vi "hash action stack.vi"(6 "init size":i32=50, 7 "stack action":T2, 8 "hash action list":T1[](array[typedef]), 9 "hash action":T1, 11 "command stack":T1[](array[typedef])) -> (1 "cursor window action out":T1, 2 "stack is empty ?":bool, 3 "command stack out":T1[](array[typedef]))   [LabVIEW 2017]
uses:
  stack action -- control.ctl
  hash action control.ctl
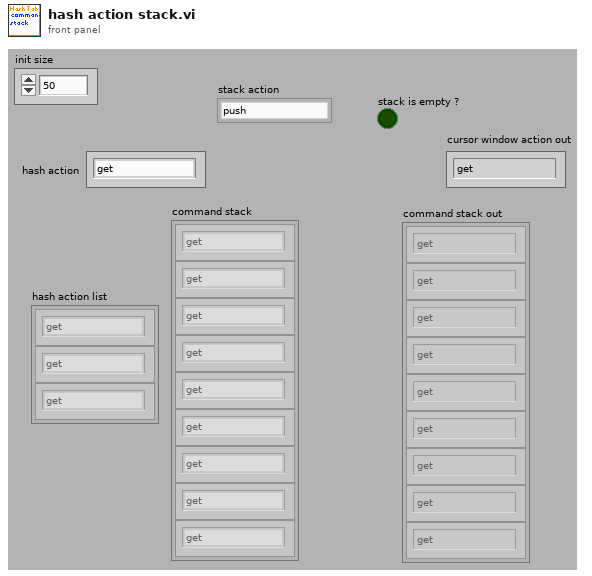
[diagram p1: front panel]
types:
  T1 = typedef "hash action control.ctl" = enum16{"get", "new", "--void", "delete", "delete all", "set", "--delete if exists", "--create if not there", "list keys", "index forw", "index back", "check", "index set", "find key"}
  T2 = typedef "stack action -- control.ctl" = enum16{"push", "pop", "check", "init"}
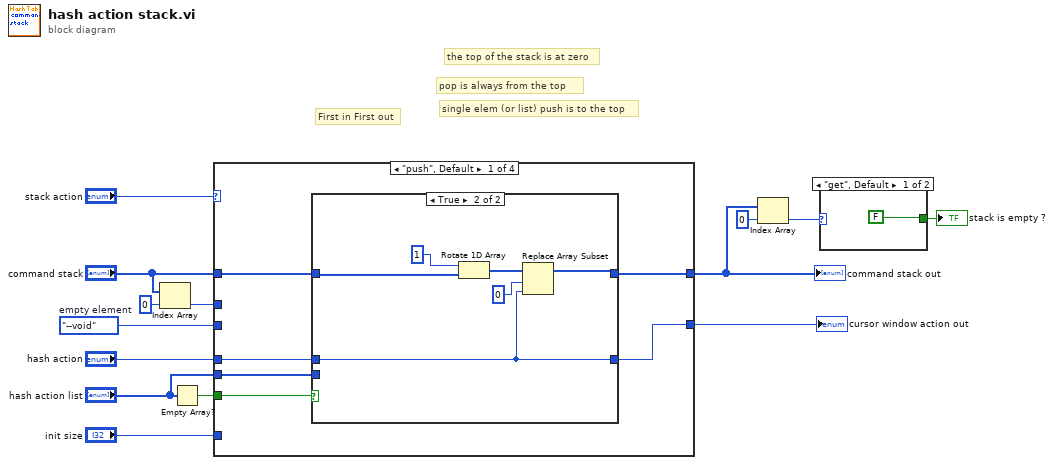
[diagram p0: block diagram]
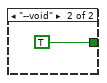
[diagram p2: hidden frame]
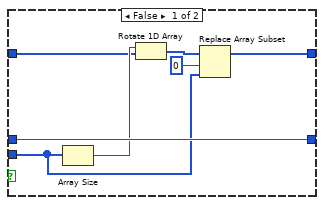
[diagram p3: hidden frame]
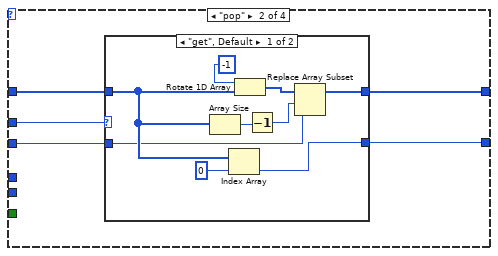
[diagram p4: hidden frame]
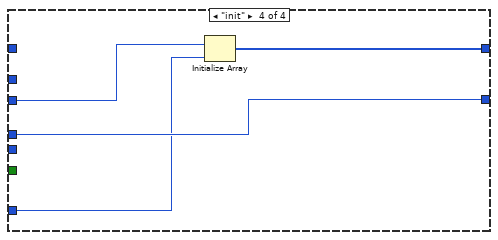
[diagram p7: hidden frame]
diagram:
  w2 = hash_action_control."--void"  # empty element
  # "single elem (or list) push is to the top"
  # "pop is always from the top"
  # "First in First out"
  # "the top of the stack is at zero"
  n1 = Index Array(array="command stack", index=0) -> (element=w6:T1)
  n2 = Empty Array?(array="hash action list") -> (empty?=w11:bool)
  n3 = case shown="\"push\", Default" "stack action" {
    tunnel: w6 -> [_ w38 _ _]
    tunnel: [w17 w37 w51 w55] -> w12
    tunnel: "hash action" -> [w20 _ w51 w55]
    tunnel: w11 -> [w19 _ _ _]
    tunnel: "hash action list" -> [w18 _ _ _]
    tunnel: "command stack" -> [w16 w36 w50 _]
    tunnel: [w15 w35 w50 w52] -> w4
    tunnel: w2 -> [_ w34 _ w54]
    tunnel: "init size" -> [_ _ _ w53]
    frame "push", Default {
      n4 = case shown="True" w19 {
        tunnel: w20 -> [w27 w31]
        tunnel: w18 -> [w21 _]
        tunnel: [w27 w31] -> w17
        tunnel: w16 -> [w23 w29]
        tunnel: [w22 w28] -> w15
        frame False {
          n5 = Array Size(array=w21) -> (size(s)=w26:i32)
          n6 = Rotate 1D Array(1:w23, 2:w26) -> (0:w25:T1[])
          n7 = Replace Array Subset(array=w25, new element=w21, index=0) -> (w22:T1[])
        }
        frame True {
          n8 = Rotate 1D Array(1:w29, 2:1) -> (0:w33:T1[])
          n9 = Replace Array Subset(array=w33, new element=w31, index=0) -> (w28:T1[])
        }
      }
    }
    frame "pop" {
      n10 = case shown="\"get\", Default" w38 {
        tunnel: [w45 w48] -> w37
        tunnel: w36 -> [w44 w49]
        tunnel: [w42 w49] -> w35
        tunnel: w34 -> [w39 w48]
        frame "get", Default {
          n11 = Array Size(array=w44) -> (size(s)=w41:i32)
          n12 = Index Array(array=w44, index=0) -> (element=w45:T1)
          n13 = Rotate 1D Array(1:w44, 2:-1) -> (0:w43:T1[])
          n14 = Decrement(x=w41) -> (x-1=w40:i32)
          n15 = Replace Array Subset(array=w43, new element=w39, index=w40) -> (w42:T1[])
        }
        frame "--void" {
        }
      }
    }
    frame "check" {
    }
    frame "init" {
      n16 = Initialize Array(w54, w53) -> (w52:T1[])
    }
  }
  "command stack out" <- w4
  "cursor window action out" <- w12
  n17 = Index Array(array=w4, index=0) -> (element=w3:T1)
  n18 = case shown="\"get\", Default" w3 {
    tunnel: [FALSE TRUE] -> w7
    frame "get", Default {
    }
    frame "--void" {
    }
  }
  "stack is empty ?" <- w7
